vi "DSF.Engine.Interface.Builder.New.vi"(7 "fifo depths (10)":u32=10, 8 "error in (no error)":errorcluster, 10 "error size (512 B)":T1=enum."512-byte", 11 "Builder Interface type":refnum<class "DSF.Engine.Interface.Builder.lvclass">) -> (0 "error out":errorcluster, 3 "Builder Interface":refnum<class "DSF.Engine.Interface.Builder.lvclass">)   [LabVIEW 2017, in "DSF.Engine.lvlib" / "DSF.Engine.Interface.Builder.lvclass"]
uses:
  DSF.Engine.Interface.Builder.lvclass
  C:/github/data-sharing-framework/dsf core/Source/Engine/Classes/Interface/DSF.Engine.Interface.lvclass
  DSF.Engine.Interface.Error Queue.Sizes.ctl
  DSF.Engine.Interface.lvclass
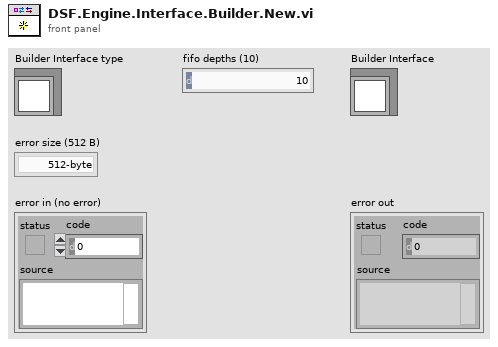
[diagram p1: front panel]
types:
  T1 = typedef "DSF.Engine.lvlib/DSF.Engine.Interface.lvclass/DSF.Engine.Interface.Error Queue.Sizes.ctl" = enum16{"256-byte", "512-byte", "1024-byte"}
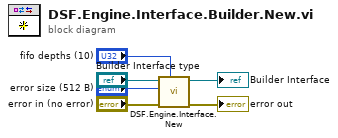
[diagram p0: block diagram]
diagram:
  n1 = call "DSF.Engine.Interface.New.vi"("fifo/queue depths (10)"="fifo depths (10)", "error in (no error)"="error in (no error)", "error size (512 B)"="error size (512 B)", "Interface type"="Builder Interface type") -> ("error out"=→"error out":errorcluster, "Interface"=→"Builder Interface":refnum<class "DSF.Engine.Interface.Builder.lvclass">)  [unwired: 6 in]
